vi "Write Parameters.vi"(8 "error in (no error)":errorcluster, 10 "Parameters":T1[](array[typedef]) {"Base Word" format="%04d"; "Address" format="%04x"; "Mask" format="%04x"; "Value" format="%016x"}, 11 "Filter in":refnum<class "Filter.lvclass">) -> (0 "error out":errorcluster, 3 "Filter out":refnum<class "Filter.lvclass">)   [LabVIEW 2020, in "BCI-1553 API.lvlib" / "Filter.lvclass"]
uses:
  Filter.lvclass
  Frames & Messages/TypeDefs/Parameter Table Data.ctl
  Frames & Messages/TypeDefs/Scaling Information.ctl
  Filter.lvclass/Filter.ctl
  BCI-1553 API.lvlib
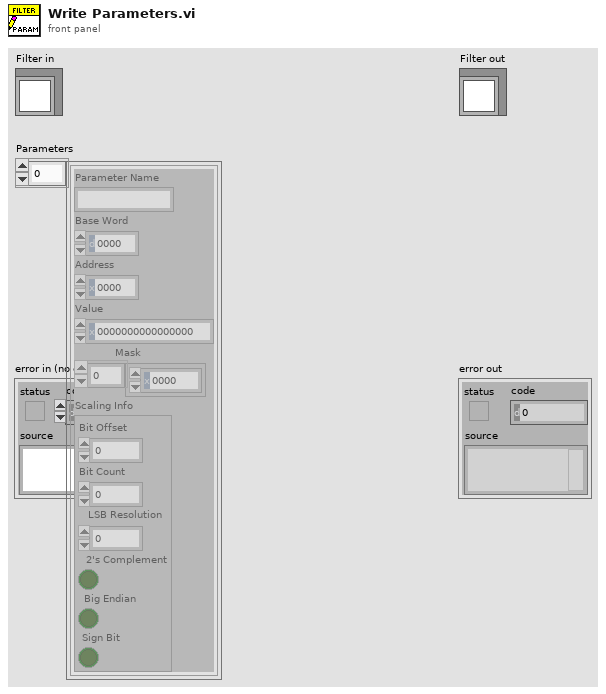
[diagram p1: front panel]
types:
  T1 = typedef "BCI-1553 API.lvlib/Parameter Table Data.ctl" = cluster{"Parameter Name":string, "Base Word":u16, "Address":u16, "Value":u64, "Mask":u16[], "Scaling Info":T2}
  T2 = typedef "BCI-1553 API.lvlib/Scaling Information.ctl" = cluster{"Bit Offset":i32, "Bit Count":i32, "LSB Resolution":dbl, "2's Complement":bool, "Big Endian":bool, "Sign Bit":bool}
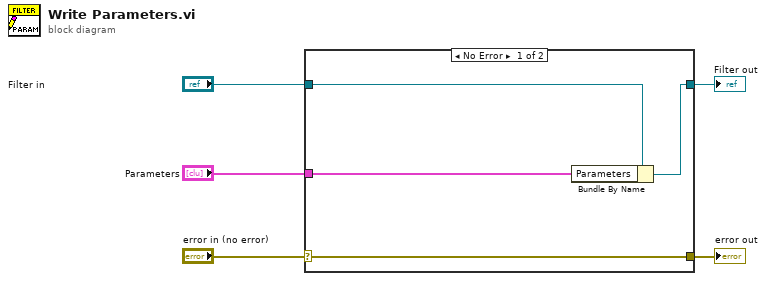
[diagram p0: block diagram]
diagram:
  n1 = case shown="No Error" "error in (no error)" {
    selector: "error in (no error)" -> [w9 w10]
    tunnel: [w9 w10] -> w4
    tunnel: [w7 w11] -> w2
    tunnel: "Filter in" -> [w8 w11]
    tunnel: "Parameters" -> [w6 _]
    frame No Error {
      n2 = Bundle By Name(cluster=w8, "Parameters"=w6) -> (w7:refnum<class "Filter.lvclass">)
    }
    frame Error {
    }
  }
  "error out" <- w4
  "Filter out" <- w2
